vi "Handle Command.vi"(8 "error in (no error)":errorcluster, 10 "CMD in":refnum<class "Update Housekeeping.lvclass">, 11 "Object In":refnum<class>) -> (0 "error out":errorcluster, 1 "Command Successful?":bool, 2 "CMD out":refnum<class "Update Housekeeping.lvclass">, 3 "Object Out":refnum<class>)   [LabVIEW 2014, in "eCRDS Library.lvlib" / "Update Housekeeping.lvclass"]
doc: "This VI will contain the code used to actually execute the request. If the request is successful, this will be indicated by the boolean output <b>Command Successful?</b>. The boolean output can then be used by the <b>Command Reply</b> which sends a reply if the reply queue is valid."
uses:
  Update Housekeeping.lvclass
  reusable/CRDS/Main/CRDS.lvclass
  Update Housekeeping.lvclass/Update Housekeeping.ctl
  reusable/CRDS/Main/CRDS.lvclass/CRDS.ctl
  reusable/CRDS/Cell/CRDS Cell.lvclass/CRDS Cell.ctl
  reusable/CRDS/Cell/Write P.vi
  reusable/CRDS/Cell/Write Q.vi
  reusable/CRDS/Cell/Write T.vi
  reusable/CRDS/Main/Write Qpurge.vi
  reusable/CRDS/Main/Read Cells.vi
  reusable/CRDS/Main/Write Cells.vi
  reusable/CRDS/Cell/CRDS Cell.lvclass
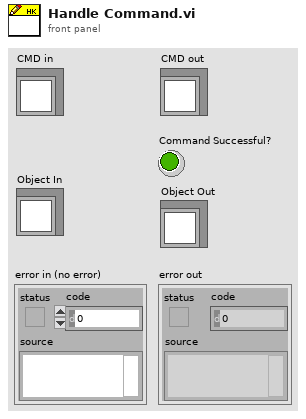
[diagram p1: front panel]
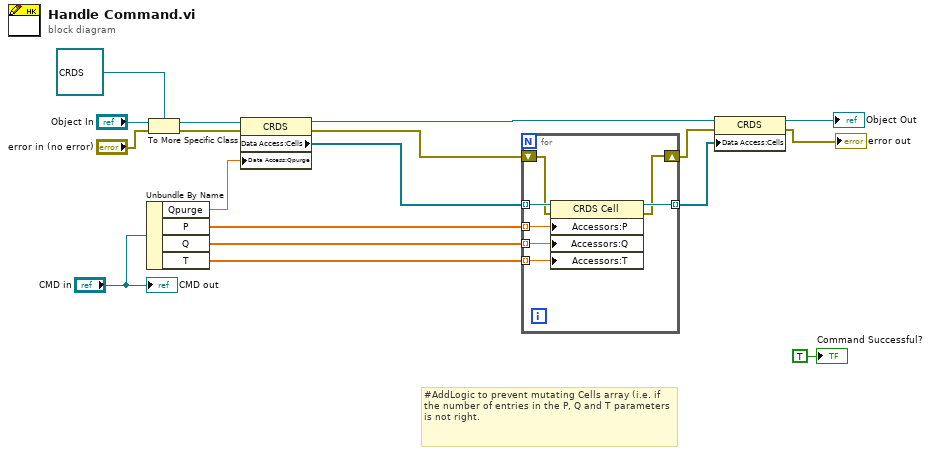
[diagram p0: block diagram]
diagram:
  # "#AddLogic to prevent mutating Cells array (i.e. if the number of entries in the P, Q and T parameters is not right."
  n1 = Unbundle By Name("CMD in") -> ("Qpurge"=w2:dbl, "P"=w10:dbl[], "Q"=w9:dbl[], "T"=w1:dbl[])
  n2 = To More Specific Class(target class=refnum<class "CRDS.lvclass"> refnum ("CRDS"), reference="Object In", error in="error in (no error)") -> (specific class reference=w15:refnum<class "CRDS.lvclass">, error out=w14:errorcluster)
  n3 = property class="CRDS"(reference=w15, error in=w14, "Data Access:Qpurge"=w2) -> (reference out=w7:refnum<class "CRDS.lvclass">, error out=w6:errorcluster, "Data Access:Cells"=w11:refnum<class "CRDS Cell.lvclass">[])
  n4 = for {
    tunnel: w1 -> [w24] mode=indexing
    tunnel: w11 -> [w25] mode=indexing
    tunnel: w10 -> [w23] mode=indexing
    tunnel: w9 -> [w22] mode=indexing
    tunnel: [w21] -> w8 mode=indexing
    shift-right: [w19] -> w5
    shift-left: w6 -> [w20]
    n5 = property class="CRDS Cell"(reference=w25, error in=w20, "Accessors:P"=w23, "Accessors:Q"=w22, "Accessors:T"=w24) -> (reference out=w21:refnum<class "CRDS Cell.lvclass">, error out=w19:errorcluster)
  }
  n6 = property class="CRDS"(reference=w7, error in=w5, "Data Access:Cells"=w8) -> (reference out=→"Object Out":refnum<class "CRDS.lvclass">, error out=→"error out":errorcluster)
  "CMD out" <- "CMD in"
  "Command Successful?" <- TRUE ("Command Successful?")
